vi "Helbako CAN.vi"(6 "Split-timer":bool, 8 "Error IN":errorcluster, 11 "CMD":u16) -> (0 "Error OUT":errorcluster)   [LabVIEW 2019]
uses:
  Type Defs/CAN Mode.ctl
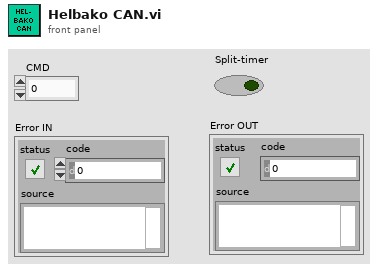
[diagram p1: front panel]
types:
  T1 = typedef "CAN Mode.ctl" = enum16{"Init", "Read", "Write", "Close"}
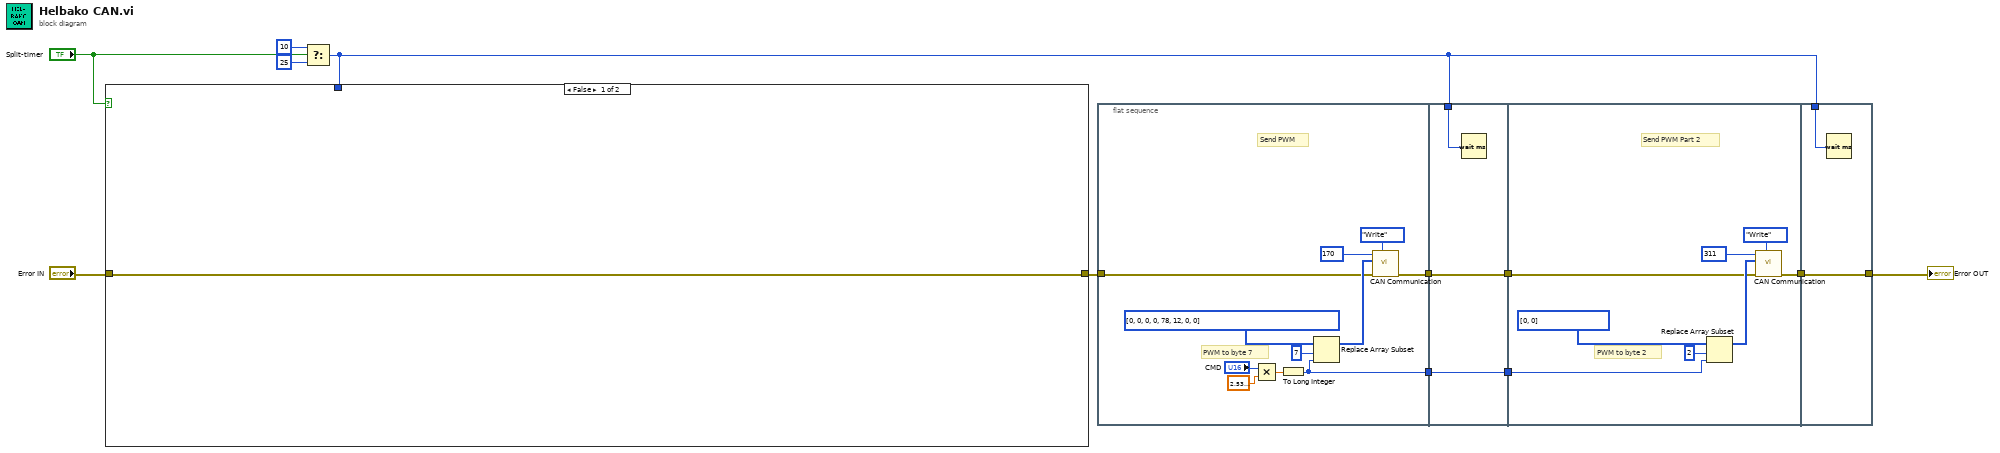
[diagram p0: block diagram]
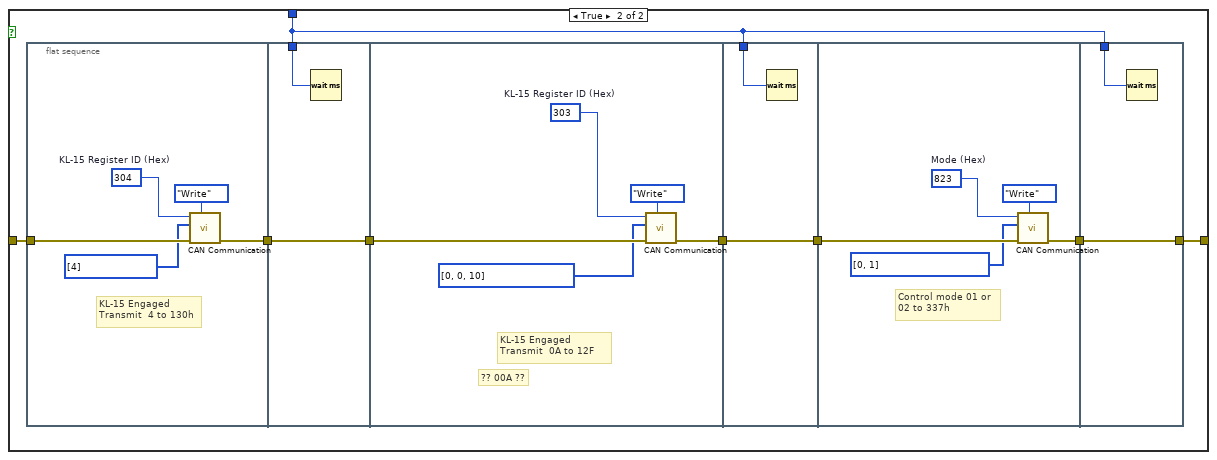
[diagram p2: hidden frame]
diagram:
  n1 = Select(t=u32 10 ("milliseconds to wait"), s="Split-timer", f=u32 25 ("milliseconds to wait")) -> (s? t:f=w3:u32)
  n2 = case shown="False" "Split-timer" {
    tunnel: "Error IN" -> [w13 w16]
    tunnel: w3 -> [_ w14]
    tunnel: [w13 w15] -> w5
    frame False {
    }
    frame True {
      n3 = flat-sequence {
        tunnel: [w25] -> w21
        tunnel: w16 -> [w24]
        tunnel: w14 -> [w28]
        tunnel: [w27] -> w20
        tunnel: w21 -> [w27]
        tunnel: w20 -> [w32]
        tunnel: [w31] -> w19
        tunnel: w14 -> [w35]
        tunnel: [w34] -> w18
        tunnel: w19 -> [w34]
        tunnel: w18 -> [w39]
        tunnel: [w38] -> w17
        tunnel: w14 -> [w42]
        tunnel: w17 -> [w41]
        tunnel: [w41] -> w15
        frame #0 {
          w23 = 304  # KL-15 Register ID (Hex)
          # "KL-15 Engaged\nTransmit  4 to 130h"
          n4 = call "CAN Communication.vi"("CAN Mode"=CAN_Mode."Write", "Error IN"=w24, "Message"=u8[] [4] ("Data Array  Constant"), "Arbitration ID"=w23) -> ("Error OUT"=w25:errorcluster)  [unwired: 6 in, 1 out]
        }
        frame #1 {
          n5 = Wait (ms)(milliseconds to wait=w28) -> ()  [unwired: 1 out]
        }
        frame #2 {
          w30 = 303  # KL-15 Register ID (Hex)
          # "?? 00A ??"
          # "KL-15 Engaged\nTransmit  0A to 12F"
          n6 = call "CAN Communication.vi"("CAN Mode"=CAN_Mode."Write", "Error IN"=w32, "Message"=u8[] [0, 0, 10] ("Data Array Constant"), "Arbitration ID"=w30) -> ("Error OUT"=w31:errorcluster)  [unwired: 6 in, 1 out]
        }
        frame #3 {
          n7 = Wait (ms)(milliseconds to wait=w35) -> ()  [unwired: 1 out]
        }
        frame #4 {
          w37 = 823  # Mode (Hex)
          # "Control mode 01 or 02 to 337h"
          n8 = call "CAN Communication.vi"("CAN Mode"=CAN_Mode."Write", "Error IN"=w39, "Message"=u8[] [0, 1] ("Data Array (Hex) Constant"), "Arbitration ID"=w37) -> ("Error OUT"=w38:errorcluster)  [unwired: 6 in, 1 out]
        }
        frame #5 {
          n9 = Wait (ms)(milliseconds to wait=w42) -> ()  [unwired: 1 out]
        }
      }
    }
  }
  n10 = flat-sequence {
    tunnel: [w52] -> w11
    tunnel: [w44] -> w10
    tunnel: w5 -> [w43]
    tunnel: w3 -> [w56]
    tunnel: w11 -> [w55]
    tunnel: [w55] -> w9
    tunnel: [w54] -> w8
    tunnel: w10 -> [w54]
    tunnel: w9 -> [w59]
    tunnel: [w58] -> w7
    tunnel: w8 -> [w57]
    tunnel: [w66] -> w6
    tunnel: w7 -> [w66]
    tunnel: w3 -> [w65]
    frame #0 {
      # "PWM to byte 7"
      # "Send PWM"
      n11 = Multiply(x="CMD", y=sgl 2.54) -> (x*y=w50:sgl)
      n12 = To Long Integer(number=w50) -> (32bit integer=w44:i32)
      n13 = Replace Array Subset(array=u8[] [0, 0, 0, 0, 78, 12, 0, 0] ("Data Array (Hex) Bytes  0 -> 7"), new element=w44, index=7) -> (w45:u8[])
      n14 = call "CAN Communication.vi"("CAN Mode"=CAN_Mode."Write", "Error IN"=w43, "Message"=w45, "Arbitration ID"=170 ("CAN Addres to Xmit\nSpeed CMD (Hex) 2")) -> ("Error OUT"=w52:errorcluster)  [unwired: 6 in, 1 out]
    }
    frame #1 {
      n15 = Wait (ms)(milliseconds to wait=w56) -> ()  [unwired: 1 out]
    }
    frame #2 {
      # "PWM to byte 2"
      # "Send PWM Part 2"
      n16 = Replace Array Subset(array=u8[] [0, 0] ("Data Array (Hex) Bytes  0 -> 7"), new element=w57, index=2) -> (w64:u8[])
      n17 = call "CAN Communication.vi"("CAN Mode"=CAN_Mode."Write", "Error IN"=w59, "Message"=w64, "Arbitration ID"=311 ("CAN Addres to Xmit\nSpeed CMD (Hex) 2")) -> ("Error OUT"=w58:errorcluster)  [unwired: 6 in, 1 out]
    }
    frame #3 {
      n18 = Wait (ms)(milliseconds to wait=w65) -> ()  [unwired: 1 out]
    }
  }
  "Error OUT" <- w6
